vi "Edit PPS.vi"(8 "error in":errorcluster, 10 "Sequence Context In":refnum<k7>, 11 "PPS Config In":T1={"VISA Resource"="", "Voltage Level (0.0 V)"=0.0, "CURRent Limit (0.0 A)"=0.0, "OVP LEVEL (0V)"=0.0, "Enable OVP (T: Enable)"=TRUE, "OCP LEVEL (0A)"=0.0, "Enable OCP (T: Enable)"=TRUE, "Value Out"="", "Value In"="", "Actual Voltage Level (V)"=0.0, "Actual Current Limit (A)"=0.0, "Select Instrument"="", "Enable Output"=FALSE, "PPS Operation"=enum."Close", "Type"=0} {"Type" items=["Voltage", "Current"]; "Actual Current Limit (A)" format="%.2f"; "Actual Voltage Level (V)" format="%.2f"; "OCP LEVEL (0A)" format="%.2f"; "OVP LEVEL (0V)" format="%.2f"; "Voltage Level (0.0 V)" format="%.2f"}) -> (0 "error out":errorcluster, 2 "Report Text":string, 3 "PPS Config Out":T1={"VISA Resource"="", "Voltage Level (0.0 V)"=0.0, "CURRent Limit (0.0 A)"=0.0, "OVP LEVEL (0V)"=0.0, "Enable OVP (T: Enable)"=TRUE, "OCP LEVEL (0A)"=0.0, "Enable OCP (T: Enable)"=TRUE, "Value Out"="", "Value In"="", "Actual Voltage Level (V)"=0.0, "Actual Current Limit (A)"=0.0, "Select Instrument"="", "Enable Output"=FALSE, "PPS Operation"=enum."Close", "Type"=0} {"Type" items=["Voltage", "Current"]; "Actual Current Limit (A)" format="%.2f"; "Actual Voltage Level (V)" format="%.2f"; "OCP LEVEL (0A)" format="%.2f"; "OVP LEVEL (0V)" format="%.2f"; "Voltage Level (0.0 V)" format="%.2f"})   [LabVIEW 2023, in "LTT_TeststandSteptypes.lvlib"]
uses:
  LTT_TeststandSteptypes.lvlib
  HardwareAbstractionLayer_LVOOP/PowerSupply/Teststand/Control/PPS StepType Control.ctl
  <vilib>/addons/TestStand/_TSUtility.llb/TestStand - Start Modal Dialog (Sequence Context).vi
  <vilib>/addons/TestStand/_TSUtility.llb/TestStand - End Modal Dialog (Sequence Context).vi
  HardwareAbstractionLayer_LVOOP/PowerSupply/PowerSupply.lvclass
panel:
  in  "Close":bool
  in  "OK":bool
  in  "PPS Operation":T2(tab)
  in  "Select Instrument":string(combo)
  in  "Current Limit (0.0 A)":dbl
  in  "Voltage Level (0.0 V)":dbl format="%.2f"
  in  "Enable OCP (T: Enable)":bool=TRUE
  in  "Enable OVP (T: Enable)":bool=TRUE
  in  "OVP LEVEL (0V)":dbl format="%.2f"
  in  "OCP LEVEL (0A)":dbl format="%.2f"
  in  "Enable Output":bool
  # "Init for Lower Power Supply\nConfiguration read from database"
  # "Self Test is Enabled by selecting this opeartion"
  # "Over Voltage Protection"
  # "Over Current Protection"
  # "Measure the  Actual Voltage and Actual Current"
  # "PPS Close Operation will be executing by selecting this opeartion"
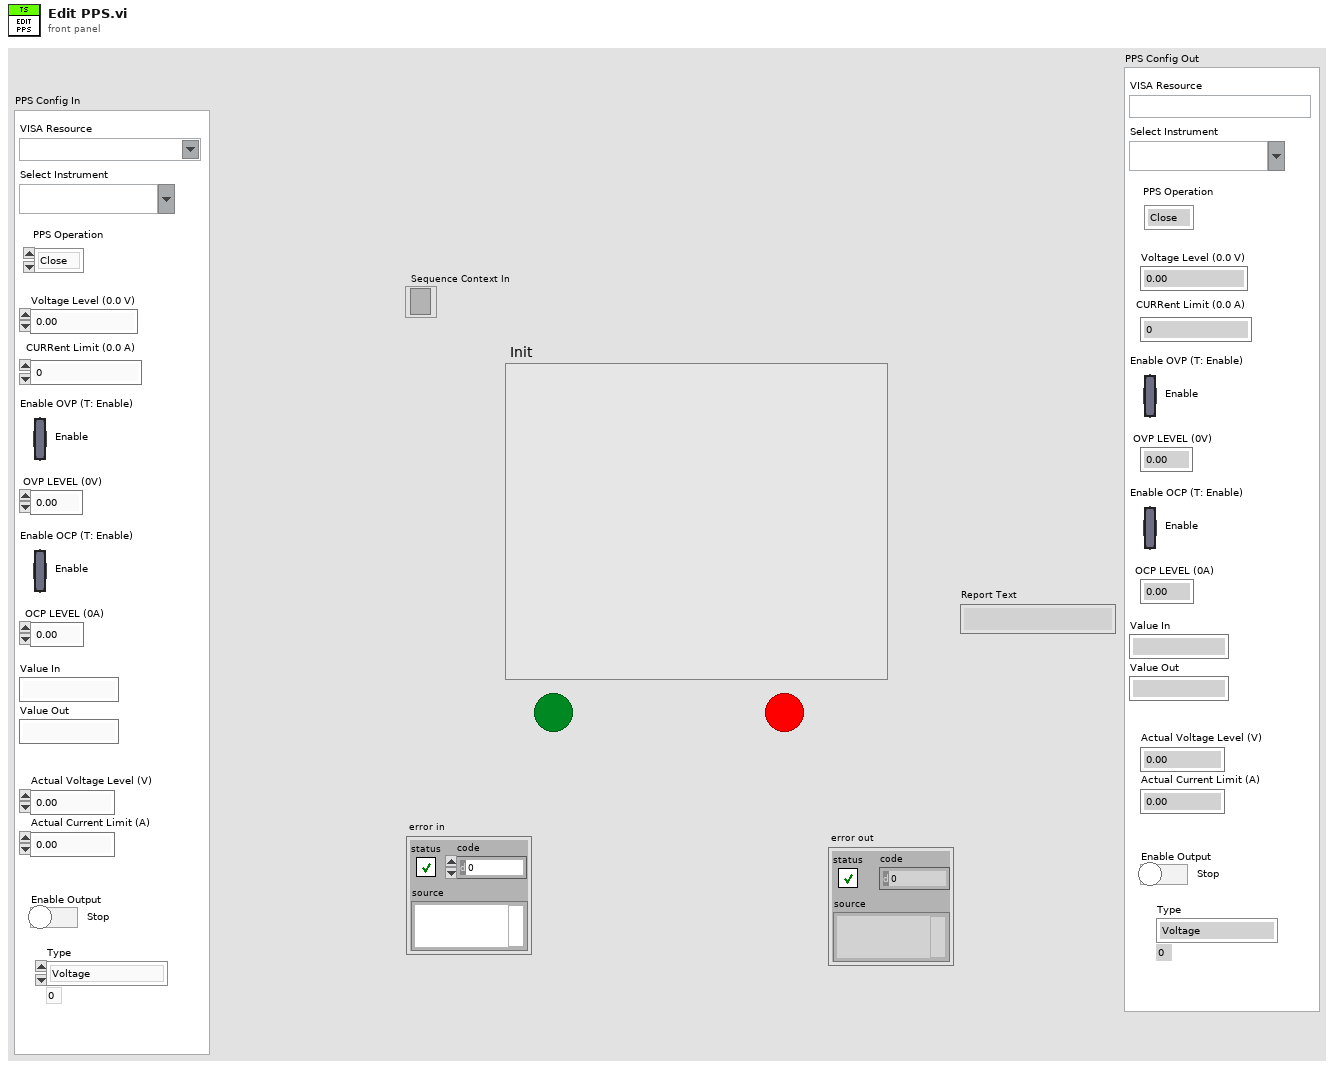
[diagram p1: front panel]
types:
  T1 = typedef "HardwareAbstractionLayer_LVOOP.lvlib/PowerSupply.lvclass/PPS StepType Control.ctl" = cluster{"VISA Resource":refnum<visa-resource-name>, "Voltage Level (0.0 V)":dbl, "CURRent Limit (0.0 A)":dbl, "OVP LEVEL (0V)":dbl, "Enable OVP (T: Enable)":bool, "OCP LEVEL (0A)":dbl, "Enable OCP (T: Enable)":bool, "Value Out":string, "Value In":string, "Actual Voltage Level (V)":dbl, "Actual Current Limit (A)":dbl, "Select Instrument":string, "Enable Output":bool, "PPS Operation":enum32{"Init", "Self Test", "Configure", "Measure", "Close"}, "Type":u16}
  T2 = enum32{"Init", "Self Test", "Configure", "Measure", "Close"}
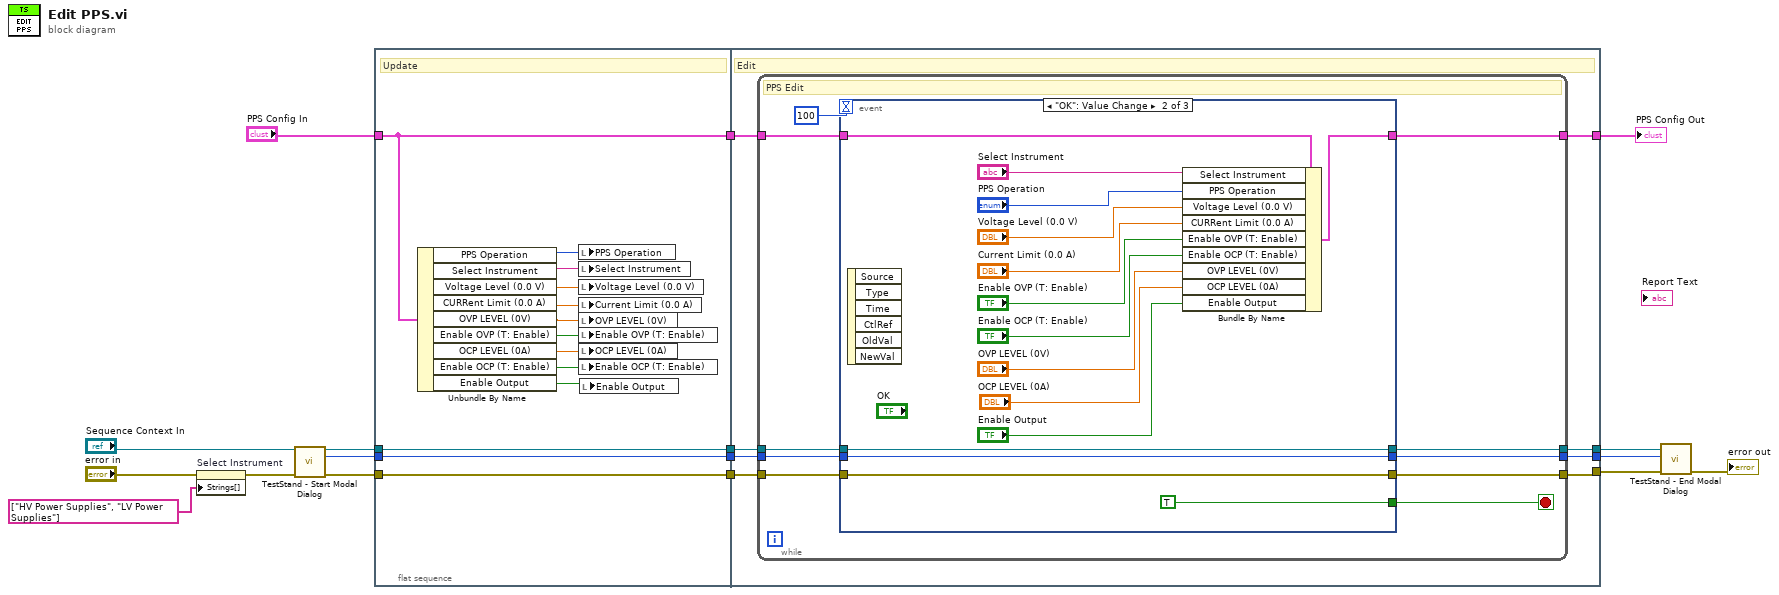
[diagram p0: block diagram]
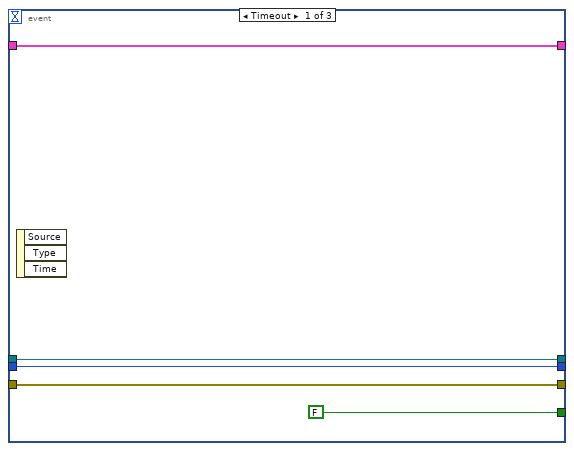
[diagram p2: hidden frame]
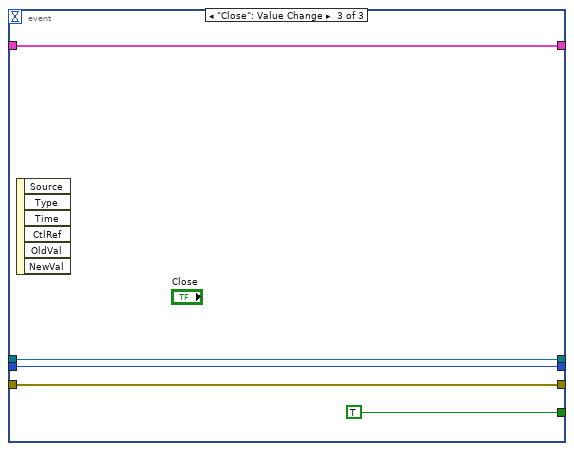
[diagram p3: hidden frame]
diagram:
  n1 = property on="Select Instrument" class="CmbBox"(error in="error in", "Strings[]"=string[] ["HV Power Supplies", "LV Power Supplies"] ("Strings []")) -> (error out=w1:errorcluster)  [unwired: 1 in, 1 out]
  n2 = call-poly <vilib>:"TestStand - Start Modal Dialog.vi"("Sequence Context In"="Sequence Context In", "error in (no error)"=w1) -> ("Sequence Context Out"=w16:refnum<k7>, "Modal ID"=w9:i32, "error out"=w15:errorcluster)  [unwired: 9 in, 2 out]
  n3 = flat-sequence {
    tunnel: w16 -> [w30]
    tunnel: w15 -> [w29]
    tunnel: [w30] -> w14
    tunnel: [w29] -> w13
    tunnel: w9 -> [w28]
    tunnel: [w28] -> w8
    tunnel: "PPS Config In" -> [w27]
    tunnel: [w27] -> w7
    tunnel: w14 -> [w36]
    tunnel: w13 -> [w38]
    tunnel: [w35] -> w12
    tunnel: [w37] -> w11
    tunnel: w8 -> [w34]
    tunnel: [w33] -> w4
    tunnel: w7 -> [w32]
    tunnel: [w31] -> w5
    frame #0 {
      # "Update"
      n4 = Unbundle By Name(w27) -> ("PPS Operation"=w26:T2, "Select Instrument"=w25:string, "Voltage Level (0.0 V)"=w24:dbl, "CURRent Limit (0.0 A)"=w23:dbl, "OVP LEVEL (0V)"=w22:dbl, "Enable OVP (T: Enable)"=w21:bool, "OCP LEVEL (0A)"=w20:dbl, "Enable OCP (T: Enable)"=w19:bool, "Enable Output"=w18:bool)
      n5 = local write "PPS Operation"(w26) -> ()
      n6 = local write "Select Instrument"(w25) -> ()
      n7 = local write "Voltage Level (0.0 V)"(w24) -> ()
      n8 = local write "Current Limit (0.0 A)"(w23) -> ()
      n9 = local write "OVP LEVEL (0V)"(w22) -> ()
      n10 = local write "Enable OVP (T: Enable)"(w21) -> ()
      n11 = local write "OCP LEVEL (0A)"(w20) -> ()
      n12 = local write "Enable OCP (T: Enable)"(w19) -> ()
      n13 = local write "Enable Output"(w18) -> ()
    }
    frame #1 {
      # "Edit"
      n14 = while {
        tunnel: w38 -> [w47]
        tunnel: [w46] -> w37
        tunnel: w36 -> [w45]
        tunnel: [w44] -> w35
        tunnel: w34 -> [w43]
        tunnel: [w42] -> w33
        tunnel: w32 -> [w40]
        tunnel: [w39] -> w31
        stop <- w41 stop-if-true
        # "PPS Edit"
        n15 = event shown="[1] \"OK\": Value Change" {
          selector: _ -> [_ _ _]
          dyn-events: _ -> [_ _ _]
          timeout: 100 -> [_ _ _]
          tunnel: w47 -> [w53 w66 w71]
          tunnel: [w53 w66 w71] -> w46
          tunnel: w45 -> [w52 w68 w73]
          tunnel: [w52 w68 w73] -> w44
          tunnel: w43 -> [w51 w67 w72]
          tunnel: [w51 w67 w72] -> w42
          tunnel: [FALSE TRUE TRUE] -> w41
          tunnel: w40 -> [w49 w64 w69]
          tunnel: [w49 w55 w69] -> w39
          event Timeout {
            n16 = event-data() -> ()  [unwired: 1 in, 3 out]
          }
          event "OK": Value Change {
            n17 = event-data() -> ()  [unwired: 1 in, 6 out]
            n18 = Bundle By Name(cluster=w64, "Select Instrument"="Select Instrument", "PPS Operation"="PPS Operation", "Voltage Level (0.0 V)"="Voltage Level (0.0 V)", "CURRent Limit (0.0 A)"="Current Limit (0.0 A)", "Enable OVP (T: Enable)"="Enable OVP (T: Enable)", "Enable OCP (T: Enable)"="Enable OCP (T: Enable)", "OVP LEVEL (0V)"="OVP LEVEL (0V)", "OCP LEVEL (0A)"="OCP LEVEL (0A)", "Enable Output"="Enable Output") -> (w55:T1)
          }
          event "Close": Value Change {
            n19 = event-data() -> ()  [unwired: 1 in, 6 out]
          }
        }
      }
    }
  }
  n20 = call-poly <vilib>:"TestStand - End Modal Dialog.vi"("Sequence Context In"=w12, "Modal ID"=w4, "error in (no error)"=w11) -> ("error out"=→"error out":errorcluster)  [unwired: 12 in]
  "PPS Config Out" <- w5
